vi "ExManualCalibWavenumbersXLSData.vi"() -> ()   [LabVIEW 2010]
uses:
  <vilib>/Utility/file.llb/Read From Spreadsheet File (DBL).vi
panel:
  in  "stop":bool
  in  "Finished picking peaks":bool
  out "XY Graph":cluster{dbl[], "first row":dbl[]}(graph)
  in  "Wavelength 3":dbl=576.96 format="%.2f"
  in  "Pixel 3":dbl=537.0 format="%.2f"
  in  "Wavelength 2":dbl=546.074 format="%.2f"
  in  "Pixel 2":dbl=485.0 format="%.2f"
  in  "Wavelength 1":dbl=435.833 format="%.2f"
  in  "Pixel 1":dbl=301.0 format="%.2f"
  out "error out":errorcluster
  in  "error in (no error)":errorcluster
  in  "Full Input File Name (include .xls extension)":path=path "C:/Program Files/SIToolKit/LabVIEW/Data Files/HG-ARGON.xls"
  # "ExManualCalibWavenumbersXLSData.vi : this example\nshows how to do a manual calibration. First select a file with\ndata in it with know peaks (i.e. mercury lamp). then start VI.\nEnter pixel of peak with what wavelength peak should be.\nThis example does three peaks, but more can be used\nif available. Once all pixels and wavelengths have been\nentered then hit the Finished button. The display will\nnow show calibrated data with wavenumbers on the \nx axis. The cursor can be moved around to verify\nthe calibration. Hit STOP button when done with calibration.\nUser may want to save calibration points in ascii file so that \nthese values can be used when collecting live data."
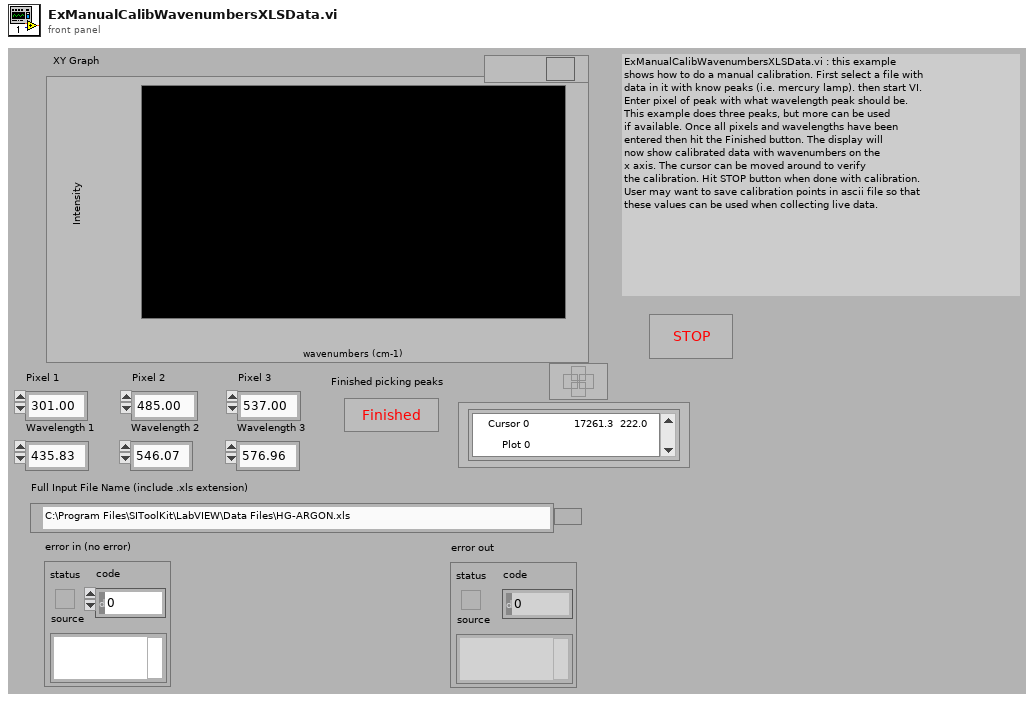
[diagram p1: front panel]
types:
  T1 = cluster{i32, "Order of\npolynominal":i32, "Input Units\n4 = wavelength in nm":i32, "Output Units\n5 = cm-1":i32, "Laser line wavelength in nm":dbl}
  T2 = cluster{"Calibrated Array":dbl[], "first row":dbl[]}
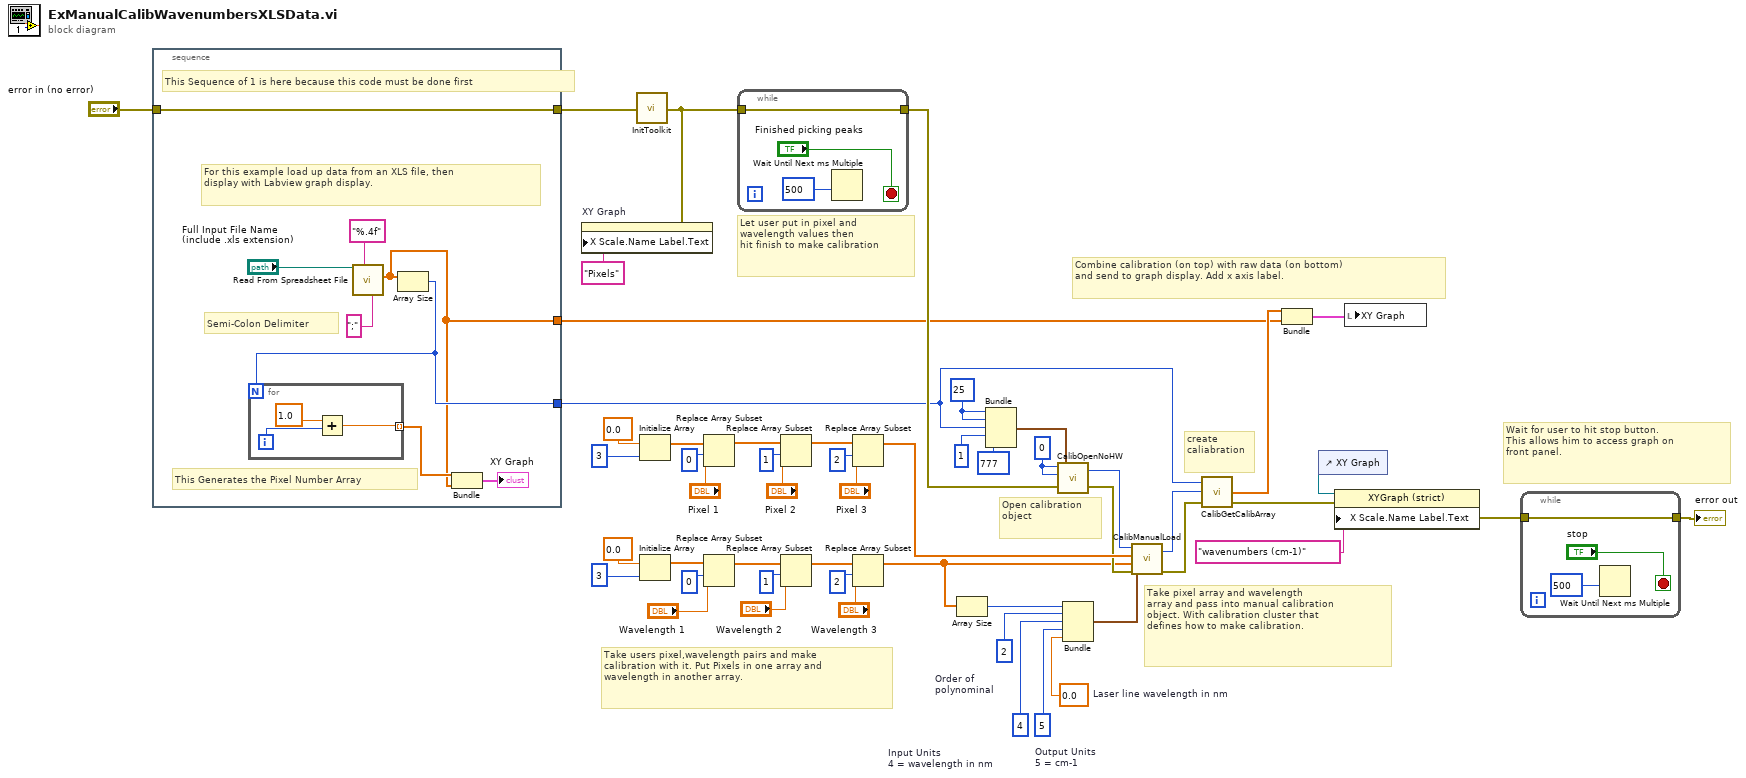
[diagram p0: block diagram]
diagram:
  w27 = 0.0  # Laser line wavelength in nm
  w28 = 5  # Output Units 5 = cm-1
  w29 = 4  # Input Units 4 = wavelength in nm
  w30 = 2  # Order of polynominal
  w31 = 0
  w33 = 25
  # "Wait for user to hit stop button.\nThis allows him to access graph on\nfront panel."
  # "Combine calibration (on top) with raw data (on bottom) \nand send to graph display. Add x axis label."
  # "create \ncaliabration"
  # "Take pixel array and wavelength \narray and pass into manual calibration \nobject. With calibration cluster that \ndefines how to make calibration."
  # "Open calibration\nobject"
  # "Take users pixel,wavelength pairs and make \ncalibration with it. Put Pixels in one array and\nwavelength in another array."
  # "Let user put in pixel and \nwavelength values then \nhit finish to make calibration"
  n1 = stacked-sequence {
    tunnel: [w58] -> w4
    tunnel: [w54] -> w3
    tunnel: "error in (no error)" -> [w56]
    tunnel: [w56] -> w1
    frame #0 {
      # "This Sequence of 1 is here because this code must be done first"
      # "This Generates the Pixel Number Array"
      # "Semi-Colon Delimiter"
      # "For this example load up data from an XLS file, then\ndisplay with Labview graph display."
      n2 = call-poly <vilib>:"Read From Spreadsheet File.vi"("delimiter (\\t)"=";", "format (%.3f)"="%.4f", "file path (dialog if empty)"="Full Input File Name (include .xls extension)") -> ("first row"=w54:dbl[])  [unwired: 4 in, 4 out]
      n3 = Array Size(array=w54) -> (size(s)=w58:i32)
      n4 = for {
        N: w58 -> [_]
        tunnel: [w62] -> w55 mode=indexing
        i -> [w63]
        n5 = Add(x=1.0, y=w63) -> (x+y=w62:dbl)
      }
      n6 = Bundle(w55, "first row"=w54) -> (→"XY Graph":cluster{dbl[], "first row":dbl[]})  [unwired: 1 in]
    }
  }
  n7 = call <userlib>:"InitToolkit.vi"("error in"=w1) -> ("error out"=w7:errorcluster)
  n8 = property on="XY Graph" class="XYGraph (strict)"(error in=w7, "X Scale.Name Label.Text"="Pixels") -> ()  [unwired: 1 in, 2 out]
  n9 = Initialize Array(0.0, 3) -> (w49:dbl[])
  n10 = Initialize Array(0.0, 3) -> (w42:dbl[])
  n11 = Replace Array Subset(array=w49, new element="Pixel 1", index=0) -> (w48:dbl[])
  n12 = Replace Array Subset(array=w42, new element="Wavelength 1", index=0) -> (w41:dbl[])
  n13 = while {
    tunnel: w7 -> [w66]
    tunnel: [w66] -> w18
    stop <- "Finished picking peaks" stop-if-true
    n14 = Wait Until Next ms Multiple(millisecond multiple=500) -> ()  [unwired: 1 out]
  }
  n15 = Replace Array Subset(array=w48, new element="Pixel 2", index=1) -> (w47:dbl[])
  n16 = Replace Array Subset(array=w41, new element="Wavelength 2", index=1) -> (w40:dbl[])
  n17 = Replace Array Subset(array=w47, new element="Pixel 3", index=2) -> (w36:dbl[])
  n18 = Replace Array Subset(array=w40, new element="Wavelength 3", index=2) -> (w6:dbl[])
  n19 = Array Size(array=w6) -> (size(s)=w5:i32)
  n20 = Bundle(w33, w33, w4, 1, 777) -> (w19:cluster{i32, i32, i32, i32, i32})  [unwired: 1 in]
  n21 = call <userlib>:"CalibOpenNoHW.vi"("error in"=w18, "Data Info"=w19, "Calibration Type"=w31, "Calibration Device ID"=w31) -> ("error out"=w34:errorcluster, "Calibration Handle"=w35:u32)
  n22 = Bundle(w5, "Order of\npolynominal"=w30, "Input Units\n4 = wavelength in nm"=w29, "Output Units\n5 = cm-1"=w28, "Laser line wavelength in nm"=w27) -> (w26:T1)  [unwired: 1 in]
  n23 = call <userlib>:"CalibManualLoad.vi"("Calibration Handle"=w35, "Pixel Array"=w36, "Wavelength Array"=w6, "error in (no error)"=w34, "Calibration Values"=w26) -> ("Calibration Handle"=w16:u32, "error out"=w17:errorcluster)
  n24 = call <userlib>:"CalibGetCalibArray.vi"("error in"=w17, "Array Size"=w4, "Calibration Handle"=w16) -> ("error out"=w13:errorcluster, "Calibrated Array"=w9:dbl[])  [unwired: 1 out]
  n25 = Bundle("Calibrated Array"=w9, "first row"=w3) -> (w15:T2)  [unwired: 1 in]
  n26 = control-ref of="XY Graph"() -> (w11:refnum<vi>)
  n27 = property on="Property Node" class="XYGraph (strict)"(reference=w11, error in=w13, "X Scale.Name Label.Text"="wavenumbers (cm-1)") -> (error out=w12:errorcluster)  [unwired: 1 out]
  n28 = local write "XY Graph"(w15) -> ()
  n29 = while {
    tunnel: w12 -> [w69]
    tunnel: [w69] -> w14
    stop <- "stop" stop-if-true
    n30 = Wait Until Next ms Multiple(millisecond multiple=500) -> ()  [unwired: 1 out]
  }
  "error out" <- w14
